vi "PLC_data read.vi"(8 "error in (no error)":errorcluster, 11 "IP Address":string[](array[string])) -> (0 "error out":errorcluster, 2 "Data":i16[][](array[numeric]), 3 "Array":errorcluster[](array[cluster]))   [LabVIEW 2017]
uses:
  <vilib>/ethernetip/ethernetip.llb/EthernetIP SLC500 Read Integer.vi
  <vilib>/ethernetip/ethernetip.lvlib
panel:
  # "INPUT"
  # "OUTPUT"
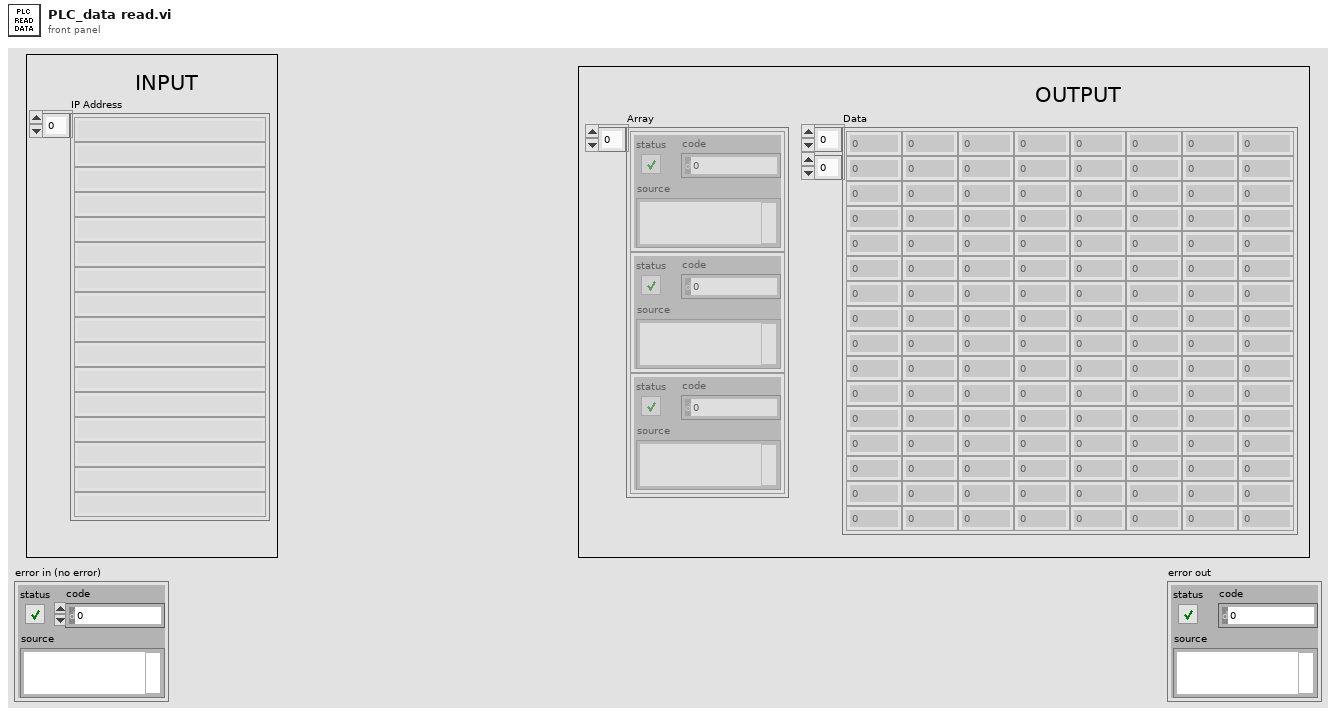
[diagram p1: front panel]
types:
  T1 = typedef "ethernetip.lvlib/ethernetip.ctl" = refnum<k21>
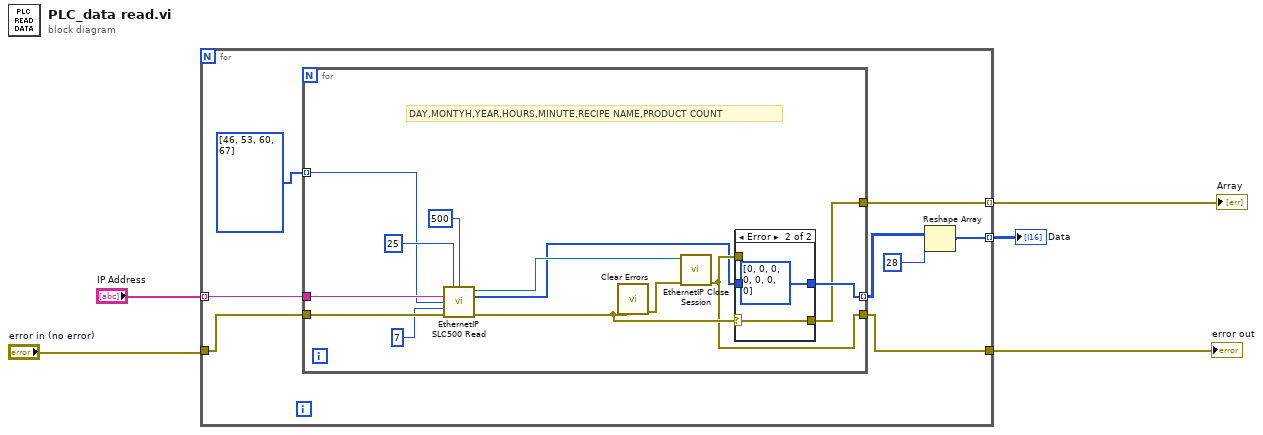
[diagram p0: block diagram]
diagram:
  n1 = for {
    tunnel: [w12] -> w4 mode=indexing
    tunnel: [w7] -> w3 mode=indexing
    tunnel: "IP Address" -> [w11] mode=indexing
    tunnel: "error in (no error)" -> [w10]
    tunnel: [w13] -> w5
    n2 = for {
      tunnel: [w15] -> w13
      tunnel: w10 -> [w26]
      tunnel: w11 -> [w25]
      tunnel: [w18] -> w8 mode=indexing
      tunnel: [w16] -> w12
      tunnel: u16[] [46, 53, 60, 67] ("Element Number") -> [w21] mode=indexing
      # "DAY,MONTYH,YEAR,HOURS,MINUTE,RECIPE NAME,PRODUCT COUNT"
      n3 = call-poly <vilib>:"EthernetIP SLC500 Read.vi"("File Number"=u16 25, "Timeout (ms)"=500, "Network Path"=w25, "Element Number"=w21, "Number of Elements"=u32 7, "error in"=w26) -> ("Session out"=w22:T1, "Data"=w14:i16[], "error out"=w17:errorcluster)  [unwired: 7 in]
      n4 = call <vilib>:"Clear Errors.vi"("error in (no error)"=w17) -> ("error out"=w19:errorcluster)  [unwired: 5 in, 1 out]
      n5 = call <vilib>:"EthernetIP Close Session.vi"("error in"=w19, "Session in"=w22) -> ("error out"=w15:errorcluster)  [unwired: 9 in]
      n6 = case shown="Error" w17 {
        selector: w17 -> [w28 w29]
        tunnel: [w28 w29] -> w16
        tunnel: [w27 i16[] [0, 0, 0, 0, 0, 0, 0] ("Data")] -> w18
        tunnel: w14 -> [w27 _]
        tunnel: w15 -> [_ _]
        frame No Error {
        }
        frame Error {
        }
      }
    }
    n7 = Reshape Array(w8, 28 ("dimension size")) -> (w7:i16[])
  }
  "Data" <- w3
  "error out" <- w5
  "Array" <- w4
